vi "test-kalman-filter.vi"(8 "error in (no error)":errorcluster) -> (0 "error out":errorcluster, 3 "ALL TESTS PASSED":bool)   [LabVIEW 2019]
uses:
  <vilib>/Rock Robotics/WPI/ThirdParty/JAS_Junk/TrajLib/LINEAR_SYSTEM.ctl
  <vilib>/Analysis/Matrix/Datatypes/RealMatrix.ctl
  <vilib>/Rock Robotics/WPI/ThirdParty/JAS_Junk/TrajLib/KALMAN_FILTER.ctl
  <vilib>/Rock Robotics/WPI/ThirdParty/JAS_Junk/TrajLib/Rotation2d_CreateAngle.vi
  <vilib>/Rock Robotics/WPI/ThirdParty/JAS_Junk/TrajLib/Translation2d_Create.vi
  <vilib>/Rock Robotics/WPI/ThirdParty/JAS_Junk/TrajLib/MatrixHelper_CoerceSize.vi
  <vilib>/Analysis/1siggen.llb/Gaussian White Noise.vi
  <vilib>/Analysis/Matrix/Numeric/Subtract/Subtract - RM,RM.vi
  <vilib>/Analysis/Matrix/Numeric/Add/Add - RM,RM.vi
  <vilib>/Rock Robotics/WPI/ThirdParty/JAS_Junk/TrajLib/Trajectory_Library.lvlib
  <vilib>/Analysis/Matrix/NI_Matrix.lvlib
panel:
  out "xHat1":dbl
  out "xHat0":dbl
  out "WhiteNoise":T1
  out "Error 3C":bool
  out "KalFilt Error 3B":bool
  out "KalFilt Error 3A":bool
  out "Test 1 Passed":bool
  out "max value 4B":dbl
  out "max value 4A":dbl
  out "Test 4 Passed":bool
  out "xHat 4":cluster{dbl[], dbl[]}(graph)
  out "Measurements 4":cluster{dbl[], dbl[]}(graph)
  out "Error 4A":bool
  out "Error 4B":bool
  out "KalFilt Error 4":errorcluster
  out "KalFilt Test 4":T2
  out "max value 3B":dbl
  out "max value 3A":dbl
  out "Test 3 Passed":bool
  out "xHats 3":cluster{dbl[], dbl[]}(graph)
  out "Measurements 3":cluster{dbl[], dbl[]}(graph)
  out "Error 3A":bool
  out "Error 3B":bool
  out "KalFilt Error 3":errorcluster
  out "KalFilt Test 3":T2
  out "Test 2 Passed":bool
  out "xHat 2":cluster{dbl[], dbl[]}(graph)
  out "Measurements 2":cluster{dbl[], dbl[]}(graph)
  out "Error 2B":bool
  out "Error 2A":bool
  out "KalFilt Error 2":errorcluster
  out "KalFilt Test 2":T2
  out "KalFilt Error 1":errorcluster
  out "KalFilt Test1":T2
  out "SwervObservError":bool
  out "SwervObservSystem":T3
  out "EllevError":bool
  out "ElevatorSystem":T3
  # "KALMAN FILTER"
  # "Steady State Gain  \n<States,Outputs>"
  # "State Estimate <Statess,1>"
  # "<States,States>"
  # "<States,Inputs>"
  # "<Outputs,States>"
  # "<Outputs,Inputs>"
  # "Steady State Gain  \n<States,Outputs>"
  # "State Estimate <Statess,1>"
  # "<States,States>"
  # "<States,Inputs>"
  # "<Outputs,States>"
  # "<Outputs,Inputs>"
  # "Steady State Gain  \n<States,Outputs>"
  # "State Estimate <Statess,1>"
  # "<States,States>"
  # "<States,Inputs>"
  # "<Outputs,States>"
  # "<Outputs,Inputs>"
  # "Steady State Gain  \n<States,Outputs>"
  # "State Estimate <Statess,1>"
  # "<States,States>"
  # "<States,Inputs>"
  # "<Outputs,States>"
  # "<Outputs,Inputs>"
  # "<States,States>"
  # "<States,Inputs>"
  # "<Outputs,States>"
  # "<Outputs,Inputs>"
  # "<States,States>"
  # "<States,Inputs>"
  # "<Outputs,States>"
  # "<Outputs,Inputs>"
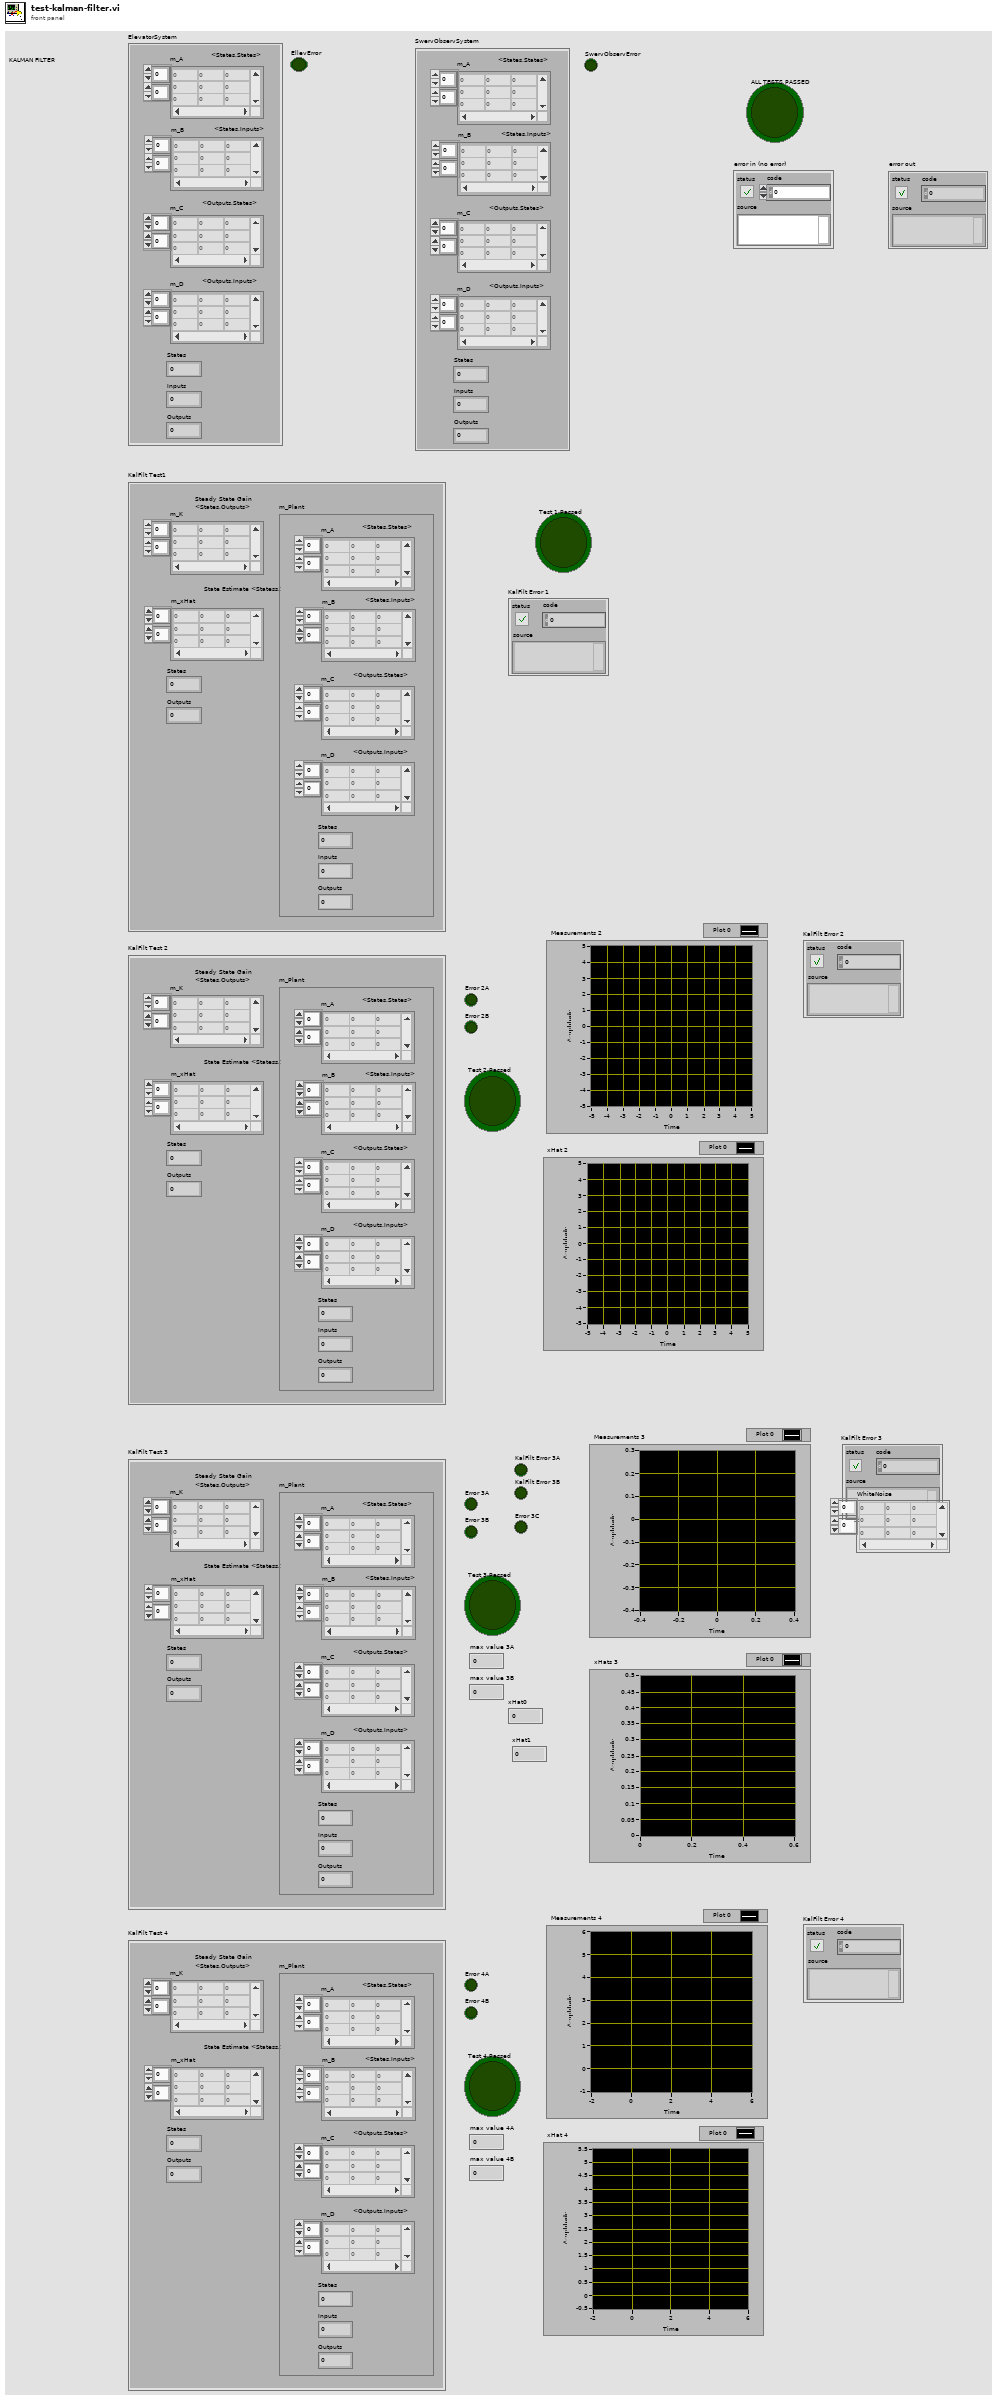
[diagram p1: front panel]
types:
  T1 = typedef "NI_Matrix.lvlib/RealMatrix.ctl" = dbl[][]
  T2 = typedef "Trajectory_Library.lvlib/KALMAN_FILTER.ctl" = cluster{"m_K":T1, "m_xHat":T1, "States":i32, "Outputs":i32, "m_Plant":T3}
  T3 = typedef "Trajectory_Library.lvlib/LINEAR_SYSTEM.ctl" = cluster{"m_A":T1, "m_B":T1, "m_C":T1, "m_D":T1, "States":i32, "Inputs":i32, "Outputs":i32}
  T4 = typedef "Trajectory_Library.lvlib/TRAJ_CONFIG.ctl" = cluster{"MaxVelocity":dbl, "Max Acceleration":dbl, "StartVelocity":dbl, "End Velocity":dbl, "Reversed":bool, "DiffDrKineConstntDefined":bool, "CentAcellConstntDefined":bool, "DiffDrVoltConstntDefined":bool, "DIFF_DRIVE_KINE_CONSTRAINT":T5, "CENTRIPETAL_ACCEL_CONSTRAINT":T7, "SwerveDrKineConstntDefined":bool, "SWERVE_DRIVE_KINE_CONSTRAINT":T8, "DIFF_DRIVE_VOLTAGE_CONSTRAINT":T11, "MECANUM_DRIVE_KINE_CONSTRAINT":T13, "MecanumDrKineConstntDefined":bool}
  T5 = typedef "Trajectory_Library.lvlib/TRAJ_CONSTRAINT_DIIF_DRIVE_KINEMATICS.ctl" = cluster{"Max Speed (M/S)":dbl, "DIFF_DRIVE_KINEMATICS":T6, "Max Accel (M/S2)":dbl}
  T6 = typedef "Trajectory_Library.lvlib/DIFF_DRIVE_KINEMATICS.ctl" = cluster{"TrackWidth_Meters":dbl}
  T7 = typedef "Trajectory_Library.lvlib/TRAJ_CONSTRAINT_CENTRIPETAL_ACCEL.ctl" = cluster{"Max Cent Accel":dbl}
  T8 = typedef "Trajectory_Library.lvlib/TRAJ_CONSTRAINT_SWERVE_DRIVE_KINEMATICS.ctl" = cluster{"Max Speed (M/S)":dbl, "SwerveKinematics":T9}
  T9 = typedef "Trajectory_Library.lvlib/SWERVE_DRIVE_KINEMATICS.ctl" = cluster{"NumModules":i32, "InverseKinematics":T1, "ForwardKinematics":T1, "Modules":T10[], "PrevCoR":T10}
  T10 = typedef "Trajectory_Library.lvlib/TRANSLATION2D.ctl" = cluster{"X":dbl, "Y":dbl}
  T11 = typedef "Trajectory_Library.lvlib/TRAJ_CONSTRAINT_DIIF_DRIVE_VOLTAGE.ctl" = cluster{"Max Voltage":dbl, "DIFF_DRIVE_KINEMATICS":T6, "SIMPLE_MOTOR_FF":T12}
  T12 = typedef "Trajectory_Library.lvlib/SIMPLE_MOTOR_FF.ctl" = cluster{"Ks":dbl, "Kv":dbl, "Ka":dbl}
  T13 = typedef "Trajectory_Library.lvlib/TRAJ_CONSTRAINT_MECA_DRIVE_KINEMATICS.ctl" = cluster{"Max Speed (M/S)":dbl, "MECA_DRIVE_KINEMATICS":T14}
  T14 = typedef "Trajectory_Library.lvlib/MECA_DRIVE_KINEMATICS.ctl" = cluster{"FrontLeft":T10, "FrontRight":T10, "RearLeft":T10, "RearRight":T10, "InverseKinematics":T1, "ForwardKinematics":T1, "PrevCoR":T10}
  T15 = typedef "Trajectory_Library.lvlib/POSE2D.ctl" = cluster{"TRANSLATION":T10, "ROTATION":T16}
  T16 = typedef "Trajectory_Library.lvlib/ROTATION2D.ctl" = cluster{"VALUE":dbl, "COS":dbl, "SIN":dbl}
  T17 = typedef "Trajectory_Library.lvlib/TRAJECTORY.ctl" = cluster{"TotalTImeSecs":dbl, "States":T18[]}
  T18 = typedef "Trajectory_Library.lvlib/TRAJ_STATE.ctl" = cluster{"TimeSeconds":dbl, "Velocity":dbl, "Acceleration":dbl, "POSE":T15, "Curvature":dbl}
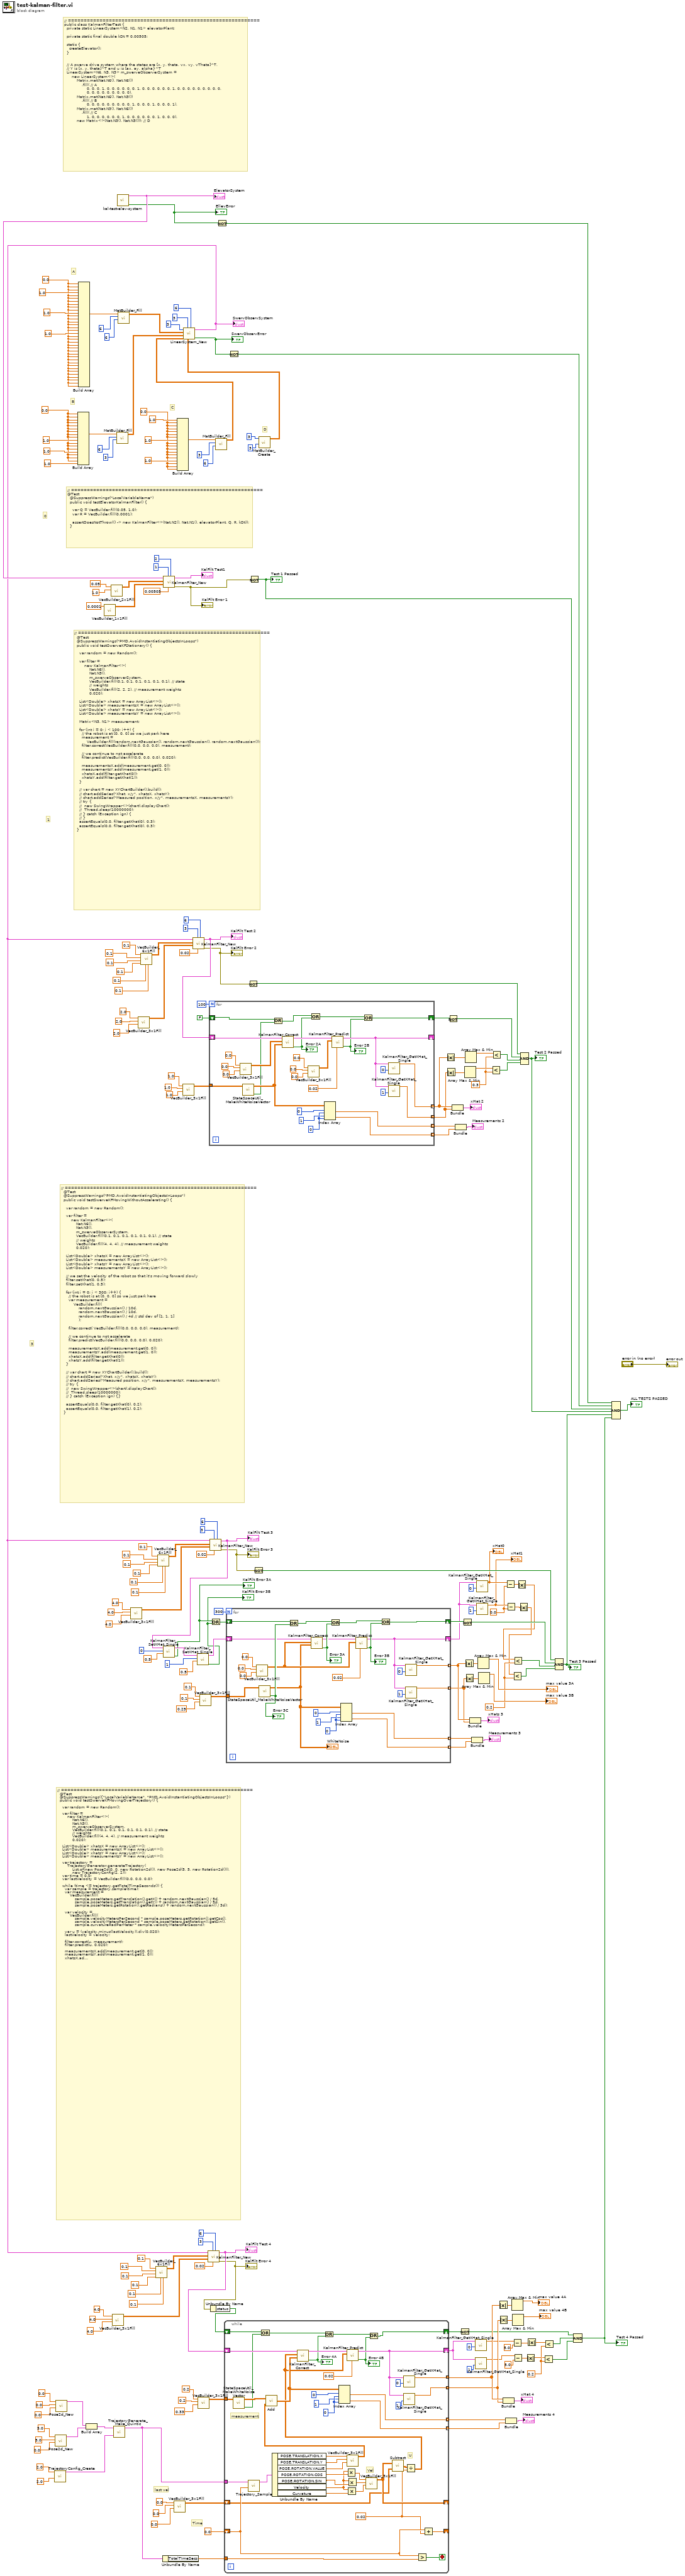
[diagram p0: block diagram]
diagram:
  w8 = 0.0
  w72 = 0.2 ("y")
  w110 = 0.2 ("y")
  w142 = 0.3 ("y")
  w189 = 0.0 ("element")
  w196 = 0.0 ("element")
  w204 = 0.0 ("element")
  # "3"
  # "1"
  # "0"
  # "last vel"
  # "Time"
  # "// =============================================================\n  @Test\n  @SuppressWarnings(\"PMD.AvoidInstantiatingObjectsInLoops\")\n  public void testSwerveKFMovingWithoutAccelerating() {\n\n    var random = new Random();\n\n    var filter =\n        new KalmanFilter<>(\n            Nat.N6(),\n            Nat.N3(),\n            m_swerveObserverSystem,\n            VecBuilder.fill(0.1, 0.1, 0.1, 0.1, 0.1, 0.1), // state\n            // weights\n            VecBuilder.fill(4, 4, 4), // measurement weights\n            0.020);\n\n    List<Double> xhatsX = new ArrayList<>();\n    List<Double> measurementsX = new ArrayList<>();\n    List<Double> xhatsY = new ArrayList<>();\n    List<Double> measurementsY = new ArrayList<>();\n\n    // we set the velocity of the robot so that it's moving forward slowly\n    filter.setXhat(0, 0.5);\n    filter.setXhat(1, 0.5);\n\n    for (int i = 0; i < 300; i++) {\n      // the robot is at [0, 0, 0] so we just park here\n      var measurement =\n          VecBuilder.fill(\n              random.nextGaussian() / 10d,\n              random.nextGaussian() / 10d,\n              random.nextGaussian() / 4d // std dev of [1, 1, 1]\n              );\n\n      filter.correct( VecBuilder.fill(0.0, 0.0, 0.0), measurement);\n\n      // we continue to not accelerate\n      filter.predict(VecBuilder.fill(0.0, 0.0, 0.0), 0.020);\n\n      measurementsX.add(measurement.get(0, 0));\n      measurementsY.add(measurement.get(1, 0));\n      xhatsX.add(filter.getXhat(0));\n      xhatsY.add(filter.getXhat(1));\n    }\n\n    // var chart = new XYChartBuilder().build();\n    // chart.addSeries(\"Xhat, x/y\", xhatsX, xhatsY);\n    // chart.addSeries(\"Measured position, x/y\", measurementsX, measurementsY);\n    // try {\n    //  new SwingWrapper<>(chart).displayChart();\n    //  Thread.sleep(10000000);\n    // } catch (Exception ign) {}\n\n    assertEquals(0.0, filter.getXhat(0), 0.2);\n    assertEquals(0.0, filter.getXhat(1), 0.2);\n  }"
  # "// =============================================================\n  @Test\n  @SuppressWarnings(\"PMD.AvoidInstantiatingObjectsInLoops\")\n  public void testSwerveKFStationary() {\n\n    var random = new Random();\n\n    var filter =\n        new KalmanFilter<>(\n            Nat.N6(),\n            Nat.N3(),\n            m_swerveObserverSystem,\n            VecBuilder.fill(0.1, 0.1, 0.1, 0.1, 0.1, 0.1), // state\n            // weights\n            VecBuilder.fill(2, 2, 2), // measurement weights\n            0.020);\n\n    List<Double> xhatsX = new ArrayList<>();\n    List<Double> measurementsX = new ArrayList<>();\n    List<Double> xhatsY = new ArrayList<>();\n    List<Double> measurementsY = new ArrayList<>();\n\n    Matrix<N3, N1> measurement;\n\n    for (int i = 0; i < 100; i++) {\n      // the robot is at [0, 0, 0] so we just park here\n      measurement =\n          VecBuilder.fill(random.nextGaussian(), random.nextGaussian(), random.nextGaussian());\n      filter.correct(VecBuilder.fill(0.0, 0.0, 0.0), measurement);\n\n      // we continue to not accelerate\n      filter.predict(VecBuilder.fill(0.0, 0.0, 0.0), 0.020);\n\n      measurementsX.add(measurement.get(0, 0));\n      measurementsY.add(measurement.get(1, 0));\n      xhatsX.add(filter.getXhat(0));\n      xhatsY.add(filter.getXhat(1));\n    }\n\n    // var chart = new XYChartBuilder().build();\n    // chart.addSeries(\"Xhat, x/y\", xhatsX, xhatsY);\n    // chart.addSeries(\"Measured position, x/y\", measurementsX, measurementsY);\n    // try {\n    //  new SwingWrapper<>(chart).displayChart();\n    //  Thread.sleep(10000000);\n    // } catch (Exception ign) {\n    // }\n    assertEquals(0.0, filter.getXhat(0), 0.3);\n    assertEquals(0.0, filter.getXhat(0), 0.3);\n  }"
  # "// =============================================================\n@Test\n  @SuppressWarnings(\"LocalVariableName\")\n  public void testElevatorKalmanFilter() {\n\n    var Q = VecBuilder.fill(0.05, 1.0);\n    var R = VecBuilder.fill(0.0001);\n\n    assertDoesNotThrow(() -> new KalmanFilter<>(Nat.N2(), Nat.N1(), elevatorPlant, Q, R, kDt));\n  }"
  # "D"
  # "C"
  # "B"
  # "A"
  # "// =============================================================\npublic class KalmanFilterTest {\n  private static LinearSystem<N2, N1, N1> elevatorPlant;\n\n  private static final double kDt = 0.00505;\n\n  static {\n    createElevator();\n  }\n\n\n  // A swerve drive system where the states are [x, y, theta, vx, vy, vTheta]^T,\n  // Y is [x, y, theta]^T and u is [ax, ay, alpha}^T\n  LinearSystem<N6, N3, N3> m_swerveObserverSystem =\n      new LinearSystem<>(\n          Matrix.mat(Nat.N6(), Nat.N6())\n              .fill( // A\n                  0, 0, 0, 1, 0, 0, 0, 0, 0, 0, 1, 0, 0, 0, 0, 0, 0, 1, 0, 0, 0, 0, 0, 0, 0, 0, 0,\n                  0, 0, 0, 0, 0, 0, 0, 0, 0),\n          Matrix.mat(Nat.N6(), Nat.N3())\n              .fill( // B\n                  0, 0, 0, 0, 0, 0, 0, 0, 0, 1, 0, 0, 0, 1, 0, 0, 0, 1),\n          Matrix.mat(Nat.N3(), Nat.N6())\n              .fill( // C\n                  1, 0, 0, 0, 0, 0, 0, 1, 0, 0, 0, 0, 0, 0, 1, 0, 0, 0),\n          new Matrix<>(Nat.N3(), Nat.N3())); // D"
  # "// =============================================================\n  @Test\n  @SuppressWarnings({\"LocalVariableName\", \"PMD.AvoidInstantiatingObjectsInLoops\"})\n  public void testSwerveKFMovingOverTrajectory() {\n\n    var random = new Random();\n\n    var filter =\n        new KalmanFilter<>(\n            Nat.N6(),\n            Nat.N3(),\n            m_swerveObserverSystem,\n            VecBuilder.fill(0.1, 0.1, 0.1, 0.1, 0.1, 0.1), // state\n            // weights\n            VecBuilder.fill(4, 4, 4), // measurement weights\n            0.020);\n\n    List<Double> xhatsX = new ArrayList<>();\n    List<Double> measurementsX = new ArrayList<>();\n    List<Double> xhatsY = new ArrayList<>();\n    List<Double> measurementsY = new ArrayList<>();\n\n    var trajectory =\n        TrajectoryGenerator.generateTrajectory(\n            List.of(new Pose2d(0, 0, new Rotation2d()), new Pose2d(5, 5, new Rotation2d())),\n            new TrajectoryConfig(2, 2));\n    var time = 0.0;\n    var lastVelocity = VecBuilder.fill(0.0, 0.0, 0.0);\n\n    while (time <= trajectory.getTotalTimeSeconds()) {\n      var sample = trajectory.sample(time);\n      var measurement =\n          VecBuilder.fill(\n              sample.poseMeters.getTranslation().getX() + random.nextGaussian() / 5d,\n              sample.poseMeters.getTranslation().getY() + random.nextGaussian() / 5d,\n              sample.poseMeters.getRotation().getRadians() + random.nextGaussian() / 3d);\n\n      var velocity =\n          VecBuilder.fill(\n              sample.velocityMetersPerSecond * sample.poseMeters.getRotation().getCos(),\n              sample.velocityMetersPerSecond * sample.poseMeters.getRotation().getSin(),\n              sample.curvatureRadPerMeter * sample.velocityMetersPerSecond);\n\n      var u = (velocity.minus(lastVelocity)).div(0.020);\n      lastVelocity = velocity;\n\n      filter.correct(u, measurement);\n      filter.predict(u, 0.020);\n\n      measurementsX.add(measurement.get(0, 0));\n      measurementsY.add(measurement.get(1, 0));\n      xhatsX.add(filter.getXhat(0));\n      xhatsY.add(filter.getXhat(1));\n\n      time += 0.020;\n    }\n\n    // var chart = new XYChartBuilder().build();\n    // chart.addSeries(\"Xhat, x/y\", xhatsX, xhatsY);\n    // chart.addSeries(\"Measured position, x/y\", measurementsX, measurementsY);\n    // try {\n    //        new SwingWrapper<>(chart).displayChart();\n    //        Thread.sleep(10000000);\n    // } catch (Exception ign) {\n    // }\n\n    assertEquals(\n        trajectory.sample(trajectory.getTotalTimeSeconds()).poseMeters.getTranslation().getX(),\n        filter.getXhat(0),\n        0.2);\n    assertEquals(\n        trajectory.sample(trajectory.getTotalTimeSeconds()).poseMeters.getTranslation().getY(),\n        filter.getXhat(1),\n        0.2);\n  }\n}"
  n1 = call <vilib>:"TrajectoryConfig_Create.vi"("MaxAcceleration"=2.0, "MaxVelocity"=2.0) -> ("TRAJECTORY_CONFIG"=w57:T4)  [unwired: 9 in]
  n2 = call <vilib>:"Pose2d_New.vi"("Heading"=0.0, "Y"=5.0, "X"=5.0) -> ("out POSe"=w61:T15)  [unwired: 8 in]
  n3 = call <vilib>:"Pose2d_New.vi"("Heading"=0.0, "Y"=0.0, "X"=0.0) -> ("out POSe"=w62:T15)  [unwired: 8 in]
  n4 = Build Array(w196, w196, w196, w196, w196, w196, w196, w196, w196, 1.0 ("element"), w196, w196, w196, 1.0 ("element"), w196, w196, w196, 1.0 ("element")) -> (w201:dbl[])
  n5 = Build Array(w204, w204, w204, 1.0 ("element"), w204, w204, w204, w204, w204, w204, 1.0 ("element"), w204, w204, w204, w204, w204, w204, 1.0 ("element"), w204, w204, w204, w204, w204, w204, w204, w204, w204, w204, w204, w204, w204, w204, w204, w204, w204, w204) -> (w212:dbl[])
  n6 = Build Array(w62, w61) -> (w60:T15[])
  n7 = call <vilib>:"VecBuilder_1x1Fill.vi"("R0_C0"=0.0001) -> ("output matrix"=w175:T1)  [unwired: 10 in]
  n8 = call <vilib>:"VecBuilder_2x1Fill.vi"("R1"=1.0, "R0"=0.05) -> ("output matrix"=w176:T1)  [unwired: 9 in]
  n9 = call <vilib>:"VecBuilder_3x1Fill.vi"("R2"=4.0, "R1"=4.0, "R0"=4.0 ("R0_C0")) -> ("output matrix"=w94:T1)  [unwired: 8 in]
  n10 = call <vilib>:"TrajectoryGenerate_Make_Quintic.vi"("traj_config"=w57, "waypointPOSE"=w60) -> ("TRAJECTORY"=w54:T17)  [unwired: 8 in, 1 out]
  n11 = call <vilib>:"MatBuilder_Fill.vi"("Columns"=3, "Rows"=6, "Value List"=w201) -> ("output matrix"=w186:T1)  [unwired: 8 in]
  n12 = call "kal-test-elev-system.vi"() -> ("Error"=w35:bool, "ElevatorSystem"=w182:T3)  [unwired: 10 in]
  "ElevatorSystem" <- w182
  "EllevError" <- w35
  n13 = call <vilib>:"MatBuilder_Fill.vi"("Columns"=6, "Rows"=6, "Value List"=w212) -> ("output matrix"=w202:T1)  [unwired: 8 in]
  n14 = call <vilib>:"VecBuilder_3x1Fill.vi"("R2"=4.0, "R1"=4.0, "R0"=4.0 ("R0_C0")) -> ("output matrix"=w133:T1)  [unwired: 8 in]
  n15 = call <vilib>:"VecBuilder_3x1Fill.vi"("R2"=2.0, "R1"=2.0, "R0"=2.0 ("R0_C0")) -> ("output matrix"=w166:T1)  [unwired: 8 in]
  n16 = call <vilib>:"VecBuilder_6x1Fill.vi"("R5"=0.1, "R4"=0.1, "R3"=0.1, "R2"=0.1, "R1"=0.1, "R0"=0.1) -> ("output matrix"=w167:T1)  [unwired: 5 in]
  n17 = call <vilib>:"VecBuilder_6x1Fill.vi"("R5"=0.1, "R4"=0.1, "R3"=0.1, "R2"=0.1, "R1"=0.1, "R0"=0.1) -> ("output matrix"=w95:T1)  [unwired: 5 in]
  n18 = call <vilib>:"VecBuilder_6x1Fill.vi"("R5"=0.1, "R4"=0.1, "R3"=0.1, "R2"=0.1, "R1"=0.1, "R0"=0.1) -> ("output matrix"=w134:T1)  [unwired: 5 in]
  n19 = Unbundle By Name(w54) -> ("TotalTImeSecs"=w53:dbl)
  n20 = call <vilib>:"KalmanFilter_New.vi"("States"=2, "dt_Seconds"=0.00505, "Outputs"=1, "MeasurementStdDevs"=w175, "StateStdDevs"=w176, "Plant"=w182) -> ("Error"=w37:errorcluster, "KalmanFilter"=→"KalFilt Test1":T2)  [unwired: 4 in]
  "KalFilt Error 1" <- w37
  n21 = call <vilib>:"VecBuilder_3x1Fill.vi"("R2"=0.0, "R1"=0.0, "R0"=0.0) -> ("output matrix"=w49:T1)  [unwired: 8 in]
  n22 = Build Array(1.0 ("element"), w189, w189, w189, w189, w189, w189, 1.0 ("element"), w189, w189, w189, w189, w189, w189, 1.0 ("element"), w189, w189, w189) -> (w195:dbl[])
  n23 = call <vilib>:"VecBuilder_3x1Fill.vi"("R2"=1.0, "R1"=1.0, "R0"=1.0) -> ("output matrix"=w154:T1)  [unwired: 8 in]
  n24 = call <vilib>:"VecBuilder_3x1Fill.vi"("R2"=0.33, "R1"=0.2, "R0"=0.2) -> ("output matrix"=w83:T1)  [unwired: 8 in]
  n25 = call <vilib>:"VecBuilder_3x1Fill.vi"("R2"=0.25, "R1"=0.1, "R0"=0.1) -> ("output matrix"=w121:T1)  [unwired: 8 in]
  n26 = call <vilib>:"MatBuilder_Fill.vi"("Columns"=6, "Rows"=3, "Value List"=w195) -> ("output matrix"=w185:T1)  [unwired: 8 in]
  n27 = Not(x=w35) -> (.not. x?=w34:bool)
  n28 = Not(x=w37) -> (.not. x?=w31:bool)
  "Test 1 Passed" <- w31
  n29 = call <vilib>:"MatBuilder_Create.vi"("Columns"=3, "Rows"=3) -> ("output matrix"=w184:T1)  [unwired: 9 in]
  n30 = call <vilib>:"LinearSystem_New.vi"("States"=6, "D"=w184, "Inputs"=3, "C"=w185, "B"=w186, "A"=w202, "Outputs"=3) -> ("Size Coerced"=w33:bool, "Linearsystem"=w69:T3)  [unwired: 3 in]
  "SwervObservSystem" <- w69
  "SwervObservError" <- w33
  n31 = call <vilib>:"KalmanFilter_New.vi"("States"=6, "dt_Seconds"=0.02, "Outputs"=3, "MeasurementStdDevs"=w166, "StateStdDevs"=w167, "Plant"=w69) -> ("Error"=w30:errorcluster, "KalmanFilter"=w153:T2)  [unwired: 4 in]
  "KalFilt Test 2" <- w153
  "KalFilt Error 2" <- w30
  n32 = call <vilib>:"KalmanFilter_New.vi"("States"=6, "dt_Seconds"=0.02, "Outputs"=3, "MeasurementStdDevs"=w94, "StateStdDevs"=w95, "Plant"=w69) -> ("Error"=w2:errorcluster, "KalmanFilter"=w55:T2)  [unwired: 4 in]
  "KalFilt Test 4" <- w55
  "KalFilt Error 4" <- w2
  n33 = for {
    N: 100 -> [_]
    tunnel: w154 -> [w242]
    shift-right: [w222] -> _
    shift-left: w153 -> [w238]
    tunnel: [w226] -> w151 mode=indexing
    tunnel: [w225] -> w150 mode=indexing
    tunnel: [w220] -> w148 mode=indexing
    tunnel: [w221] -> w147 mode=indexing
    shift-right: [w219] -> w23
    shift-left: FALSE -> [w214]
    w229 = 0 ("index (col)")
    n34 = call <vilib>:"VecBuilder_3x1Fill.vi"("R2"=0.0, "R1"=0.0, "R0"=0.0) -> ("output matrix"=w237:T1)  [unwired: 8 in]
    n35 = call <vilib>:"StateSpaceUtil_MakeWhiteNoiseVector.vi"("StdDevs"=w242) -> ("Size Coerced"=w215:bool, "WhiteNoise"=w230:T1)  [unwired: 9 in]
    n36 = Or(x=w214, y=w215) -> (x .or. y?=w213:bool)
    n37 = call <vilib>:"KalmanFilter_Correct.vi"("Y"=w230, "U"=w237, "in KalmanFilter"=w238) -> ("Error"=w216:bool, "out KalmanFilter"=w233:T2)  [unwired: 7 in]
    "Error 2A" <- w216
    n38 = call <vilib>:"VecBuilder_3x1Fill.vi"("R2"=0.0, "R1"=0.0, "R0"=0.0) -> ("output matrix"=w232:T1)  [unwired: 8 in]
    n39 = Or(x=w213, y=w216) -> (x .or. y?=w218:bool)
    n40 = Index Array(array=w230, index (row) #1=0 ("index (row)"), index (col) #1=w229, index (row) #2=1 ("index (row)"), index (col) #2=w229) -> (element #1=w226:dbl, element #2=w225:dbl)
    n41 = call <vilib>:"KalmanFilter_Predict.vi"("dT_Seconds"=0.02, "U"=w232, "in KalmanFilter"=w233) -> ("Error"=w217:bool, "out KalmanFilter"=w222:T2)  [unwired: 7 in]
    "Error 2B" <- w217
    n42 = Or(x=w218, y=w217) -> (x .or. y?=w219:bool)
    n43 = call <vilib>:"KalmanFilter_GetXHat_Single.vi"("Row"=0, "in KalmanFilter"=w222) -> ("xHat"=w220:dbl)  [unwired: 9 in]
    n44 = call <vilib>:"KalmanFilter_GetXHat_Single.vi"("Row"=1, "in KalmanFilter"=w222) -> ("xHat"=w221:dbl)  [unwired: 9 in]
  }
  n45 = call <vilib>:"KalmanFilter_New.vi"("States"=6, "dt_Seconds"=0.02, "Outputs"=3, "MeasurementStdDevs"=w133, "StateStdDevs"=w134, "Plant"=w69) -> ("Error"=w29:errorcluster, "KalmanFilter"=w107:T2)  [unwired: 4 in]
  "KalFilt Test 3" <- w107
  "KalFilt Error 3" <- w29
  n46 = call <vilib>:"KalmanFilter_SetXHat_Single.vi"("xHat"=0.5, "Row"=0, "in KalmanFilter"=w107) -> ("Error"=w20:bool, "out KalmanFilter"=w106:T2)  [unwired: 7 in]
  "KalFilt Error 3A" <- w20
  n47 = call <vilib>:"KalmanFilter_SetXHat_Single.vi"("xHat"=0.5, "Row"=1, "in KalmanFilter"=w106) -> ("Error"=w19:bool, "out KalmanFilter"=w105:T2)  [unwired: 7 in]
  "KalFilt Error 3B" <- w19
  n48 = Or(x=w20, y=w19) -> (x .or. y?=w21:bool)
  n49 = Unbundle By Name(w2) -> ("status"=w1:bool)
  n50 = while {
    tunnel: w83 -> [w287]
    shift-right: [w276] -> w46
    shift-left: w55 -> [w286]
    tunnel: [w280] -> w81 mode=indexing
    tunnel: [w279] -> w80 mode=indexing
    tunnel: [w274] -> w78 mode=indexing
    tunnel: [w275] -> w77 mode=indexing
    shift-right: [w272] -> _
    shift-left: 0.0 -> [w255]
    tunnel: w54 -> [w273]
    tunnel: w53 -> [w270]
    shift-right: [w254] -> _
    shift-left: w49 -> [w253]
    shift-right: [w243] -> w15
    shift-left: w1 -> [w246]
    stop <- w271 stop-if-true
    w251 = 0.02 ("y")
    w283 = 0 ("index (col)")
    # "U"
    # "Vel"
    # "measurement"
    n51 = call <vilib>:"StateSpaceUtil_MakeWhiteNoiseVector.vi"("StdDevs"=w287) -> ("Size Coerced"=w249:bool, "WhiteNoise"=w265:T1)  [unwired: 9 in]
    n52 = call <vilib>:"Trajectory_Sample.vi"("Time"=w255, "InputTRAJECTORY"=w273) -> ("OutputTRAJ_STATE"=w269:T18)  [unwired: 9 in]
    n53 = Or(x=w246, y=w249) -> (x .or. y?=w245:bool)
    n54 = Unbundle By Name(w269) -> ("POSE.TRANSLATION.X"=w268:dbl, "POSE.TRANSLATION.Y"=w267:dbl, "POSE.ROTATION.VALUE"=w266:dbl, "POSE.ROTATION.COS"=w262:dbl, "POSE.ROTATION.SIN"=w261:dbl, "Velocity"=w260:dbl, "Curvature"=w259:dbl)
    n55 = Multiply(x=w260, y=w262) -> (x*y=w258:dbl)
    n56 = Multiply(x=w260, y=w259) -> (x*y=w256:dbl)
    n57 = Multiply(x=w260, y=w261) -> (x*y=w257:dbl)
    n58 = call <vilib>:"VecBuilder_3x1Fill.vi"("R2"=w266, "R1"=w267, "R0"=w268) -> ("output matrix"=w264:T1)  [unwired: 8 in]
    n59 = call-poly <vilib>:"Add.vi"("Real Matrix B"=w264, "Real Matrix A"=w265) -> ("A + B"=w263:T1)
    n60 = Index Array(array=w263, index (row) #1=0 ("index (row)"), index (col) #1=w283, index (row) #2=1 ("index (row)"), index (col) #2=w283) -> (element #1=w280:dbl, element #2=w279:dbl)
    n61 = call <vilib>:"VecBuilder_3x1Fill.vi"("R2"=w256, "R1"=w257, "R0"=w258) -> ("output matrix"=w254:T1)  [unwired: 8 in]
    n62 = call-poly <vilib>:"Subtract.vi"("Real Matrix B"=w253, "Real Matrix A"=w254) -> ("A - B"=w252:T1)
    n63 = Divide(x=w252, y=w251) -> (x/y=w250:T1)
    n64 = call <vilib>:"KalmanFilter_Correct.vi"("Y"=w263, "U"=w250, "in KalmanFilter"=w286) -> ("Error"=w248:bool, "out KalmanFilter"=w285:T2)  [unwired: 7 in]
    "Error 4A" <- w248
    n65 = Or(x=w245, y=w248) -> (x .or. y?=w244:bool)
    n66 = call <vilib>:"KalmanFilter_Predict.vi"("dT_Seconds"=0.02, "U"=w250, "in KalmanFilter"=w285) -> ("Error"=w247:bool, "out KalmanFilter"=w276:T2)  [unwired: 7 in]
    "Error 4B" <- w247
    n67 = Or(x=w244, y=w247) -> (x .or. y?=w243:bool)
    n68 = call <vilib>:"KalmanFilter_GetXHat_Single.vi"("Row"=0, "in KalmanFilter"=w276) -> ("xHat"=w274:dbl)  [unwired: 9 in]
    n69 = call <vilib>:"KalmanFilter_GetXHat_Single.vi"("Row"=1, "in KalmanFilter"=w276) -> ("xHat"=w275:dbl)  [unwired: 9 in]
    n70 = Greater?(x=w255, y=w270) -> (0:w271:bool)
    n71 = Add(x=w255, y=w251) -> (x+y=w272:dbl)
  }
  n72 = for {
    N: 300 -> [_]
    tunnel: w121 -> [w313]
    shift-right: [w288] -> w11
    shift-left: w105 -> [w290]
    tunnel: [w305] -> w119 mode=indexing
    tunnel: [w304] -> w118 mode=indexing
    tunnel: [w300] -> w116 mode=indexing
    tunnel: [w301] -> w115 mode=indexing
    shift-right: [w293] -> w16
    shift-left: w21 -> [w299]
    w308 = 0 ("index (col)")
    n73 = call <vilib>:"VecBuilder_3x1Fill.vi"("R2"=0.0, "R1"=0.0, "R0"=0.0) -> ("output matrix"=w292:T1)  [unwired: 8 in]
    n74 = call <vilib>:"StateSpaceUtil_MakeWhiteNoiseVector.vi"("StdDevs"=w313) -> ("Size Coerced"=w298:bool, "WhiteNoise"=w291:T1)  [unwired: 9 in]
    "Error 3C" <- w298
    "WhiteNoise" <- w291
    n75 = Or(x=w299, y=w298) -> (x .or. y?=w297:bool)
    n76 = call <vilib>:"KalmanFilter_Correct.vi"("Y"=w291, "U"=w292, "in KalmanFilter"=w290) -> ("Error"=w296:bool, "out KalmanFilter"=w289:T2)  [unwired: 7 in]
    "Error 3A" <- w296
    n77 = Or(x=w297, y=w296) -> (x .or. y?=w294:bool)
    n78 = Index Array(array=w291, index (row) #1=0 ("index (row)"), index (col) #1=w308, index (row) #2=1 ("index (row)"), index (col) #2=w308) -> (element #1=w305:dbl, element #2=w304:dbl)
    n79 = call <vilib>:"KalmanFilter_Predict.vi"("dT_Seconds"=0.02, "U"=w292, "in KalmanFilter"=w289) -> ("Error"=w295:bool, "out KalmanFilter"=w288:T2)  [unwired: 7 in]
    "Error 3B" <- w295
    n80 = Or(x=w294, y=w295) -> (x .or. y?=w293:bool)
    n81 = call <vilib>:"KalmanFilter_GetXHat_Single.vi"("Row"=0, "in KalmanFilter"=w288) -> ("xHat"=w300:dbl)  [unwired: 9 in]
    n82 = call <vilib>:"KalmanFilter_GetXHat_Single.vi"("Row"=1, "in KalmanFilter"=w288) -> ("xHat"=w301:dbl)  [unwired: 9 in]
  }
  n83 = Not(x=w33) -> (.not. x?=w32:bool)
  n84 = Not(x=w30) -> (.not. x?=w27:bool)
  n85 = Not(x=w29) -> (.not. x?=w18:bool)
  n86 = Absolute Value(x=w148) -> (abs(x)=w145:dbl[])
  n87 = Absolute Value(x=w147) -> (abs(x)=w146:dbl[])
  n88 = Not(x=w23) -> (.not. x?=w22:bool)
  n89 = Bundle(w148, w147) -> (→"xHat 2":cluster{dbl[], dbl[]})  [unwired: 1 in]
  n90 = Bundle(w151, w150) -> (→"Measurements 2":cluster{dbl[], dbl[]})  [unwired: 1 in]
  n91 = Not(x=w15) -> (.not. x?=w14:bool)
  n92 = Not(x=w16) -> (.not. x?=w17:bool)
  n93 = Absolute Value(x=w116) -> (abs(x)=w113:dbl[])
  n94 = Absolute Value(x=w115) -> (abs(x)=w114:dbl[])
  n95 = Array Max & Min(array=w146) -> (max value=w144:dbl)  [unwired: 3 out]
  n96 = Array Max & Min(array=w145) -> (max value=w143:dbl)  [unwired: 3 out]
  n97 = Bundle(w116, w115) -> (→"xHats 3":cluster{dbl[], dbl[]})  [unwired: 1 in]
  n98 = Bundle(w119, w118) -> (→"Measurements 3":cluster{dbl[], dbl[]})  [unwired: 1 in]
  n99 = call <vilib>:"KalmanFilter_GetXHat_Single.vi"("Row"=0, "in KalmanFilter"=w46) -> ("xHat"=w41:dbl)  [unwired: 9 in]
  n100 = call <vilib>:"KalmanFilter_GetXHat_Single.vi"("Row"=1, "in KalmanFilter"=w46) -> ("xHat"=w40:dbl)  [unwired: 9 in]
  n101 = call <vilib>:"KalmanFilter_GetXHat_Single.vi"("Row"=0, "in KalmanFilter"=w11) -> ("xHat"=w10:dbl)  [unwired: 9 in]
  "xHat0" <- w10
  n102 = call <vilib>:"KalmanFilter_GetXHat_Single.vi"("Row"=1, "in KalmanFilter"=w11) -> ("xHat"=w9:dbl)  [unwired: 9 in]
  "xHat1" <- w9
  n103 = Array Max & Min(array=w113) -> (max value=→"max value 3A":dbl)  [unwired: 3 out]
  n104 = Array Max & Min(array=w114) -> (max value=→"max value 3B":dbl)  [unwired: 3 out]
  n105 = Less?(x=w144, y=w142) -> (x < y?=w140:bool)
  n106 = Less?(x=w143, y=w142) -> (x < y?=w141:bool)
  n107 = Absolute Value(x=w78) -> (abs(x)=w75:dbl[])
  n108 = Absolute Value(x=w77) -> (abs(x)=w76:dbl[])
  n109 = Bundle(w78, w77) -> (→"xHat 4":cluster{dbl[], dbl[]})  [unwired: 1 in]
  n110 = Subtract(x=w10, y=w8) -> (x-y=w7:dbl)
  n111 = Subtract(x=w9, y=w8) -> (x-y=w6:dbl)
  n112 = Bundle(w81, w80) -> (→"Measurements 4":cluster{dbl[], dbl[]})  [unwired: 1 in]
  n113 = Array Max & Min(array=w75) -> (max value=→"max value 4A":dbl)  [unwired: 3 out]
  n114 = Subtract(x=w41, y=5.0) -> (x-y=w43:dbl)
  n115 = Array Max & Min(array=w76) -> (max value=→"max value 4B":dbl)  [unwired: 3 out]
  n116 = Subtract(x=w40, y=5.0) -> (x-y=w42:dbl)
  n117 = Absolute Value(x=w7) -> (abs(x)=w4:dbl)
  n118 = Less?(x=w4, y=w110) -> (x < y?=w109:bool)
  n119 = Absolute Value(x=w6) -> (abs(x)=w5:dbl)
  n120 = Less?(x=w5, y=w110) -> (x < y?=w108:bool)
  n121 = Compound Arithmetic op=AND(w27, w22, w141, w140) -> (w24:bool)
  "Test 2 Passed" <- w24
  n122 = Absolute Value(x=w42) -> (abs(x)=w44:dbl)
  n123 = Absolute Value(x=w43) -> (abs(x)=w45:dbl)
  n124 = Less?(x=w44, y=w72) -> (x < y?=w70:bool)
  n125 = Less?(x=w45, y=w72) -> (x < y?=w71:bool)
  n126 = Compound Arithmetic op=AND(w18, w17, w109, w108) -> (w25:bool)
  "Test 3 Passed" <- w25
  n127 = Compound Arithmetic op=AND(w14, w71, w70) -> (w26:bool)
  "Test 4 Passed" <- w26
  n128 = Compound Arithmetic op=AND(w34, w32, w31, w24, w25, w26) -> (→"ALL TESTS PASSED":bool)
  "error out" <- "error in (no error)"
